vi "Actor Core.vi"(8 "error in":errorcluster, 11 "DAQmx Sequencer in":refnum<class "DAQmx Sequencer.lvclass">) -> (0 "error out":errorcluster, 3 "Actor out":refnum<class "Actor.lvclass">)   [LabVIEW 2015, in "DAQmx Sequencer.lvlib" / "DAQmx Sequencer.lvclass"]
doc: "(<B>Filename</B>: Actor Framework.lvlib:Actor.lvclass:Actor Core.vi)\n\nReceives messages to the actor, reacts to them, and initiates any error handling that may shut the actor down.\n\nDescendant classes may override this VI to append parallel tasks for the actor to complete while it handles messages. Overrides use the Call Parent Method node."
uses:
  DAQmx Sequencer.lvclass
  Sequencer/Sequencer/Sequencer.lvclass
  <vilib>/ActorFramework/Actor/Actor.lvclass
  <userlib>/_Win8uiFramework/ViewableActor.lvclass
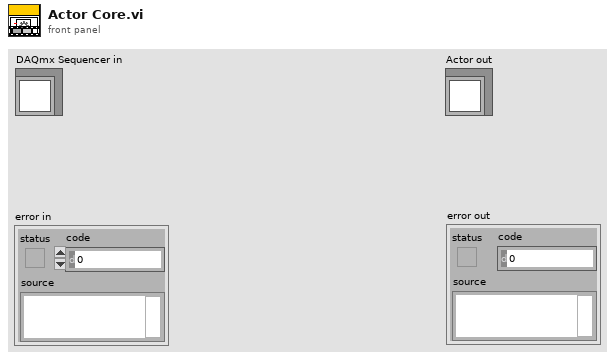
[diagram p1: front panel]
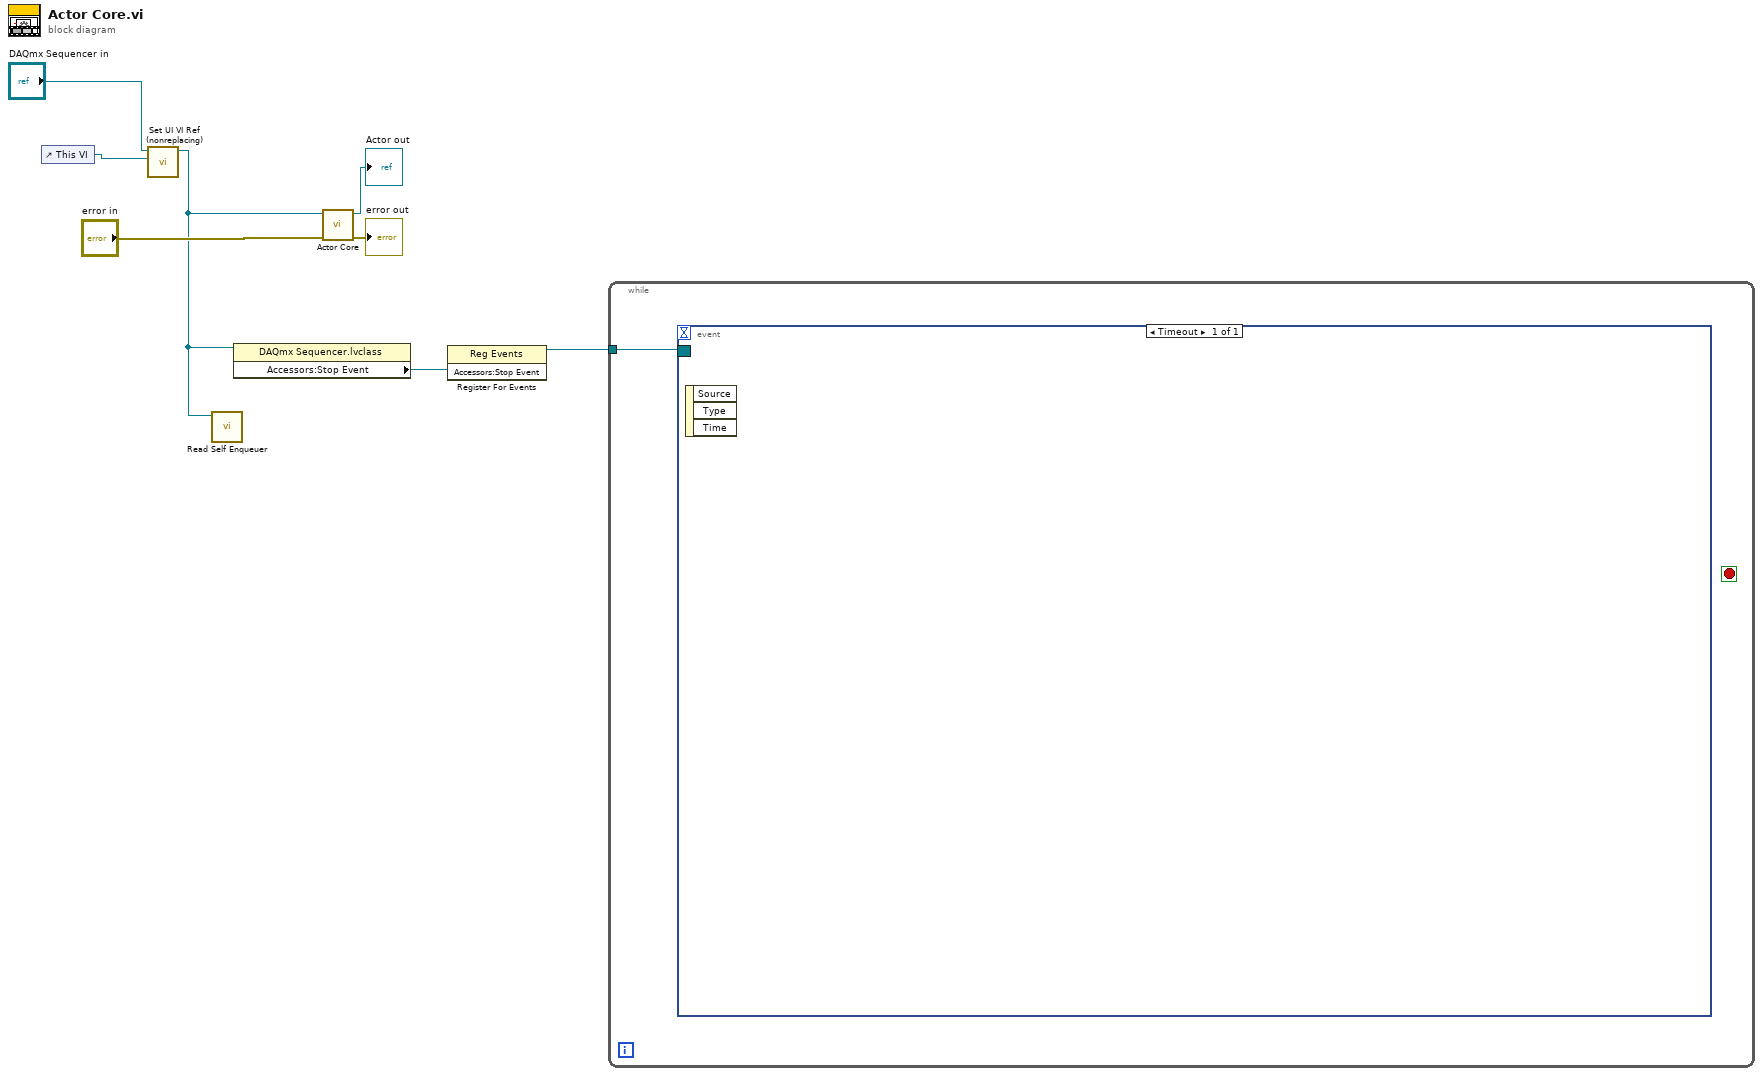
[diagram p0: block diagram]
diagram:
  n1 = control-ref of="This VI"() -> (w2:refnum<vi>)
  n2 = call <userlib>:"Set UI VI Ref (nonreplacing).vi"("UI VI Ref"=w2, "ViewableActor in"="DAQmx Sequencer in") -> ("ViewableActor out"=w3:refnum<class "DAQmx Sequencer.lvclass">)  [unwired: 7 in, 2 out]
  n3 = call <vilib>:"Read Self Enqueuer.vi"("Actor"=w3) -> ()  [unwired: 10 in, 1 out]
  n4 = property class="DAQmx Sequencer.lvclass"(reference=w3) -> ("Accessors:Stop Event"=w5:refnum<user-event>)  [unwired: 1 in, 2 out]
  n5 = call-parent "Actor Core.vi"("error in"="error in", "Sequencer in"=w3) -> ("error out"=→"error out":errorcluster, "Actor out"=→"Actor out":refnum<class "Actor.lvclass">)  [unwired: 8 in]
  n6 = register-events(w5) -> (reference out=w1:refnum<event-registration>)  [unwired: 2 in, 1 out]
  n7 = while {
    tunnel: w1 -> [w9]
    stop <- _ stop-if-true
    n8 = event shown="[0] Timeout" {
      selector: w9 -> [_]
      dyn-events: _ -> [_]
      timeout: _ -> [_]
      event Timeout {
        n9 = event-data() -> ()  [unwired: 1 in, 3 out]
      }
    }
  }
